vi "ChannelDecoder (SubVI).vi"(1 "DataArray":u32[](array[numeric])) -> (0 "Channels":u32[][](array[numeric]))   [LabVIEW 2018]
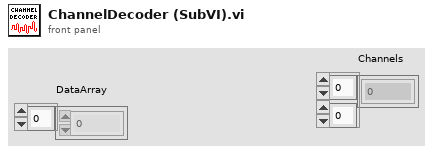
[diagram p1: front panel]
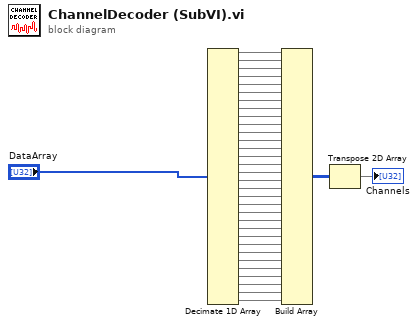
[diagram p0: block diagram]
diagram:
  n1 = Decimate 1D Array("DataArray") -> (w2:u32[], w3:u32[], w4:u32[], w5:u32[], w6:u32[], w7:u32[], w8:u32[], w9:u32[], w10:u32[], w11:u32[], w12:u32[], w13:u32[], w14:u32[], w15:u32[], w16:u32[], w17:u32[], w18:u32[], w19:u32[], w20:u32[], w21:u32[], w22:u32[], w23:u32[], w24:u32[], w25:u32[], w26:u32[], w27:u32[], w28:u32[], w29:u32[], w30:u32[], w31:u32[], w32:u32[], w33:u32[])
  n2 = Build Array(w2, w3, w4, w5, w6, w7, w8, w9, w10, w11, w12, w13, w14, w15, w16, w17, w18, w19, w20, w21, w22, w23, w24, w25, w26, w27, w28, w29, w30, w31, w32, w33) -> (w34:u32[][])
  n3 = Transpose 2D Array(2D array=w34) -> (transposed array=→"Channels":u32[][])
